vi "Track_overlay_draw_speed_test.vi"() -> ()   [LabVIEW 2018]
uses:
  <userlib>/_OpenG.lib/numeric/numeric.llb/Random Number Within Range - DBL__ogtk.vi
  Tracker.lvlib
panel:
  in  "Multiline grouping":i32=100
  out "Seconds per hour Image":dbl
  out "Image":picture
  in  "Background color Image":u32(colorbox)=13816530
  in  "Every N samples to merge":i32=2500
  out "Seconds per hour IMAQdx":dbl
  out "Image":T1(plugin-control)
  out "Error Out":errorcluster
  in  "Error In":errorcluster
  in  "Background color":u32(colorbox)=13816530
  in  "Track length, seconds (@100 fps)":i32=10
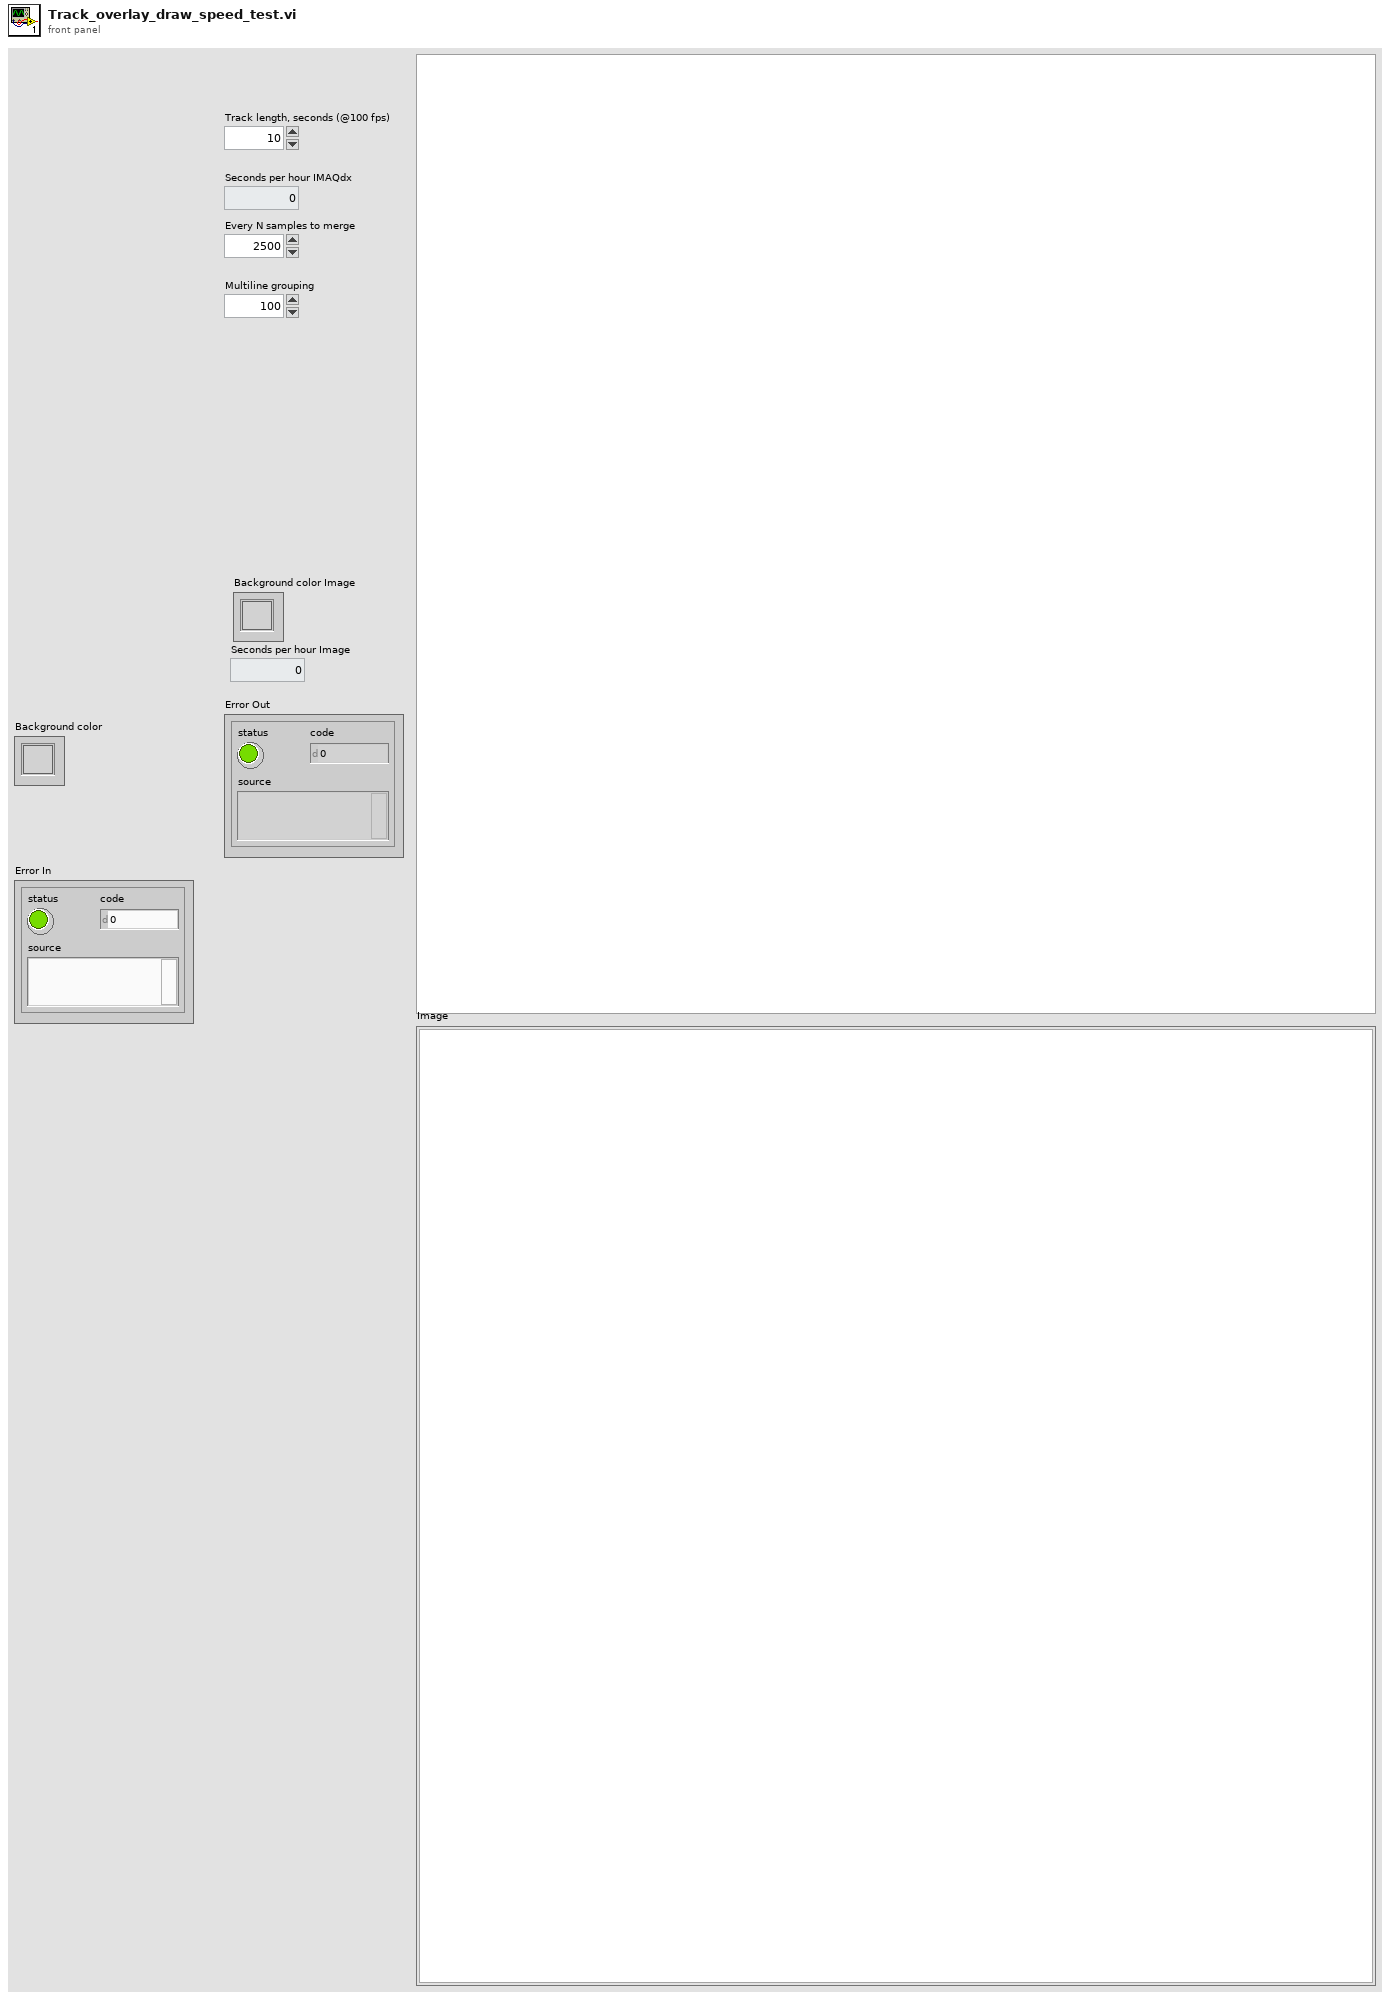
[diagram p1: front panel]
types:
  T1 = typedef "IMAQ Image.ctl" = refnum<image>
  T2 = cluster{"Left":i32, "Top":i32, "Right":i32, "Bottom":i32}
  T3 = typedef "Image Type" = u32
  T4 = cluster{"Random Number":dbl, "Random Number":dbl}
  T5 = cluster{"Random Number":dbl, "Random Number":dbl}[]
  T6 = cluster{"Width":u16, "Style":enum32{"Solid", "Dash", "Dot", "DashDot", "DashDotDot"}}
  T7 = typedef "imagedata.ctl" = cluster{"image type":i32, "image depth":i32, "image":u8[], "mask":u8[], "colors":u32[], "Rectangle":cluster{"left":i16, "top":i16, "right":i16, "bottom":i16}}
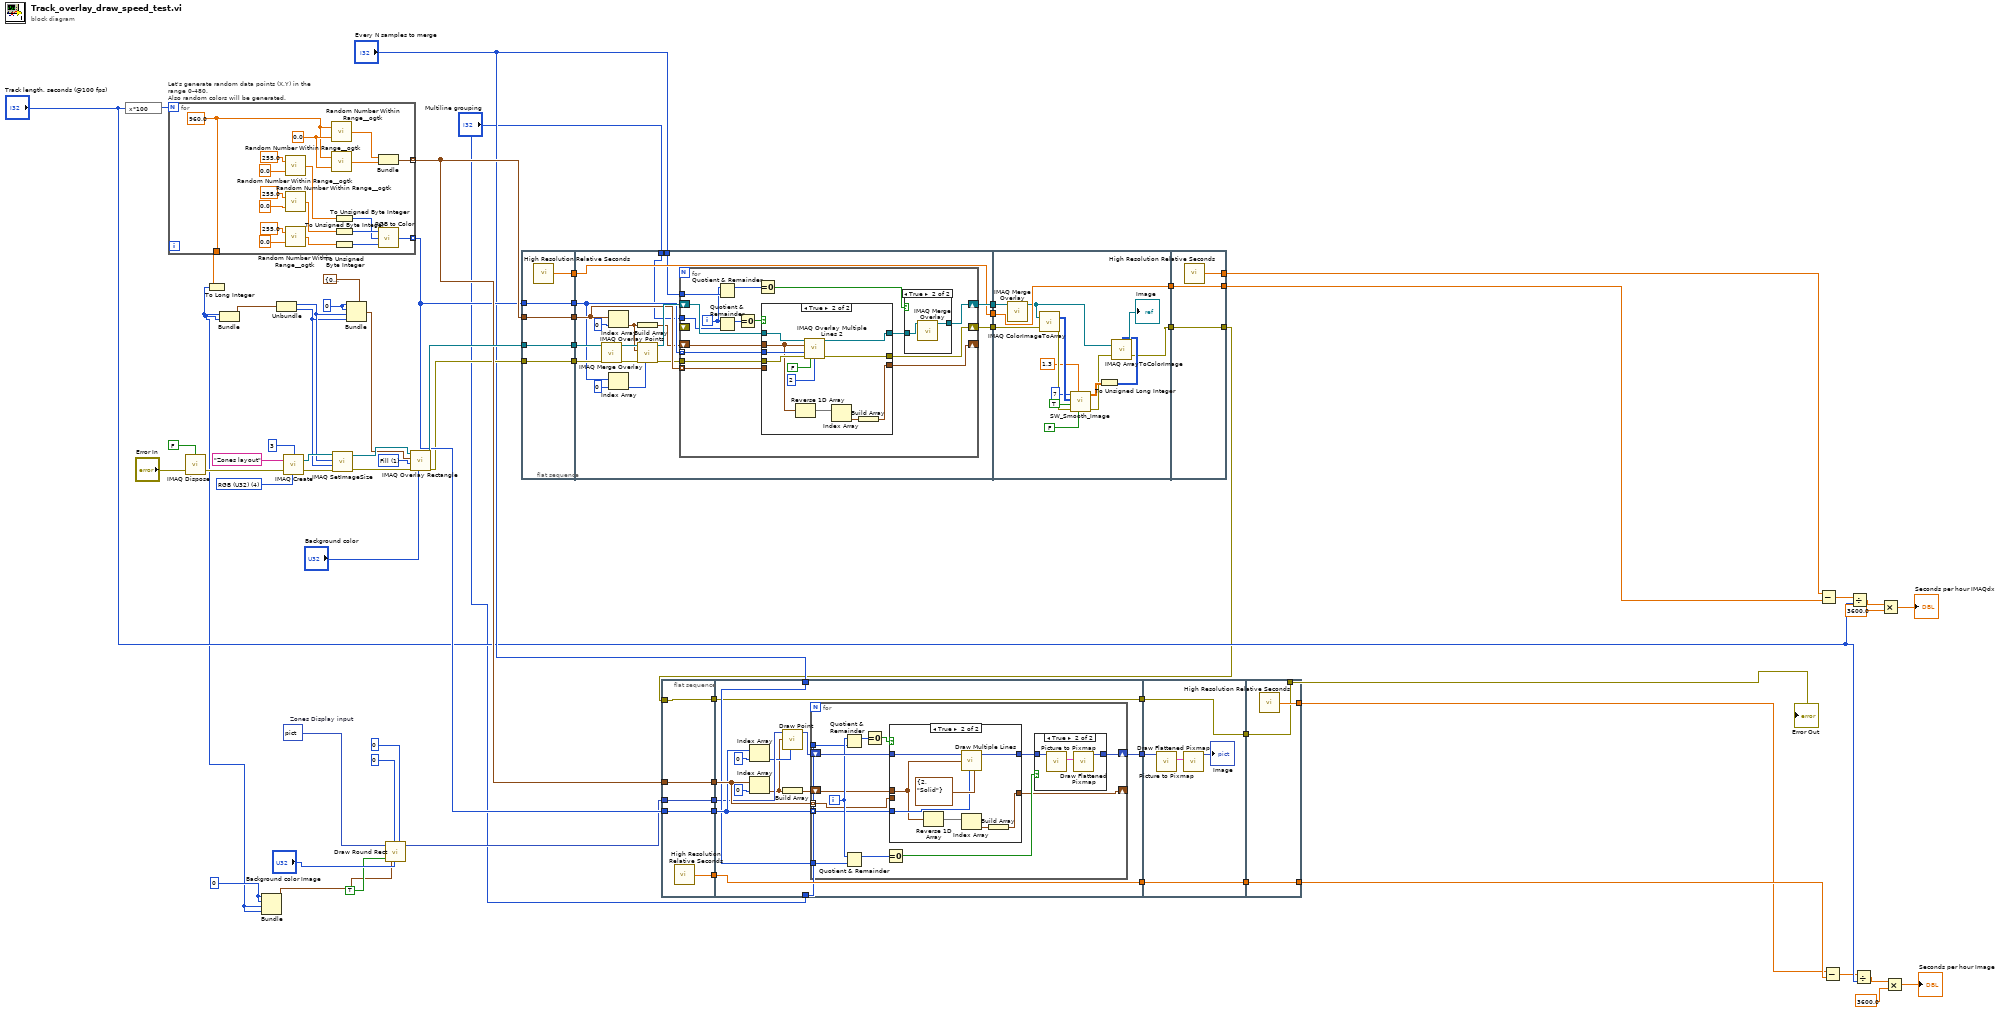
[diagram p0: block diagram]
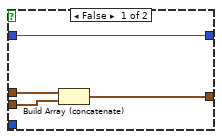
[diagram p2: hidden frame]
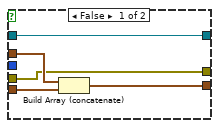
[diagram p4: hidden frame]
diagram:
  w2 = 0
  w50 = picture data[5B]  # Zones Display input
  w57 = 0 ("Left")
  w62 = u32 1 items=["Frame", "Fill", "Highlight"] ("Drawing Mode (Frame)")
  w67 = T3 4 items=["Grayscale (U8)", "Grayscale (I16)", "Grayscale (SGL)", "Complex (CSG)", "RGB (U32)", "HSL (U32)", "RGB (U64)", "Grayscale (U16)"] ("Image Type")
  n1 = expression code="x*100"("Track length, seconds (@100 fps)") -> (w70:i32)
  n2 = for "Let's generate random data points (X,Y) in the range 0-480.\nAlso random colors will be generated." {
    N: w70 -> [_]
    tunnel: [w86] -> w46 mode=indexing
    tunnel: [w72] -> w45 mode=indexing
    tunnel: [w71] -> w4
    w85 = 0.0 ("Low")
    w71 = 960.0 ("High")
    n3 = call-poly <userlib>:"Random Number Within Range__ogtk.vi"("High"=255.0, "Low"=0.0) -> ("Random Number"=w81:dbl)  [unwired: 3 in]
    n4 = call-poly <userlib>:"Random Number Within Range__ogtk.vi"("High"=255.0, "Low"=0.0) -> ("Random Number"=w80:dbl)  [unwired: 3 in]
    n5 = call-poly <userlib>:"Random Number Within Range__ogtk.vi"("High"=255.0, "Low"=0.0) -> ("Random Number"=w74:dbl)  [unwired: 3 in]
    n6 = call-poly <userlib>:"Random Number Within Range__ogtk.vi"("High"=w71, "Low"=w85) -> ("Random Number"=w88:dbl)  [unwired: 3 in]
    n7 = call-poly <userlib>:"Random Number Within Range__ogtk.vi"("High"=w71, "Low"=w85) -> ("Random Number"=w87:dbl)  [unwired: 3 in]
    n8 = To Unsigned Byte Integer(number=w81) -> (unsigned 8bit integer=w82:u8)
    n9 = To Unsigned Byte Integer(number=w80) -> (unsigned 8bit integer=w77:u8)
    n10 = To Unsigned Byte Integer(number=w74) -> (unsigned 8bit integer=w73:u8)
    n11 = Bundle("Random Number"=w88, "Random Number"=w87) -> (w86:T4)  [unwired: 1 in]
    n12 = call <vilib>:"RGB to Color.vi"("B"=w73, "G"=w77, "R"=w82) -> ("Color"=w72:u32)
  }
  n13 = call "IMAQ Dispose"("All Images? (No)"=FALSE, "error in (no error)"="Error In") -> ("error out"=w53:errorcluster)  [unwired: 4 in]
  n14 = To Long Integer(number=w4) -> (32bit integer=w1:i32)
  n15 = Bundle(w1, w1) -> (w5:cluster{i32, i32})  [unwired: 1 in]
  n16 = Bundle(w2, w2, w1, w1) -> (w3:cluster{i32, i32, i32, i32})  [unwired: 1 in]
  n17 = Unbundle(w5) -> (w59:i32, w58:i32)
  n18 = call "IMAQ Create"("Border Size"=3, "Image Name"="Zones layout", "Image Type"=w67, "error in (no error)"=w53) -> ("New Image"=w65:T1, "error out"=w66:errorcluster)  [unwired: 1 in]
  n19 = call "IMAQ SetImageSize"("error in (no error)"=w66, "Y Resolution"=w58, "X Resolution"=w59, "Image"=w65) -> ("error out"=w64:errorcluster, "Image Out"=w63:T1)  [unwired: 1 in]
  n20 = Bundle(cluster=T2 {"Left"=0, "Top"=0, "Right"=480, "Bottom"=480} ("Rectangle"), "Left"=w57, "Top"=w57, "Right"=w59, "Bottom"=w58) -> (w60:T2)
  n21 = call <vilib>:"Draw Round Rect.vi"("picture"=w50, "oval width"=i16 0, "rect"=w3, "fill?(F)"=TRUE, "color(black)"="Background color Image", "oval height"=i16 0) -> ("new picture"=w42:picture)  [unwired: 3 in]
  n22 = call "IMAQ Overlay Rectangle"("Color"="Background color", "error in (no error)"=w64, "Drawing Mode (Frame)"=w62, "Rectangle"=w60, "Image"=w63) -> ("error out"=w44:errorcluster, "Image Out"=w56:T1)  [unwired: 5 in]
  n23 = flat-sequence {
    tunnel: w45 -> [w90]
    tunnel: w46 -> [w91]
    tunnel: w44 -> [w92]
    tunnel: w56 -> [w93]
    tunnel: [w93] -> w27
    tunnel: [w92] -> w26
    tunnel: [w91] -> w25
    tunnel: [w90] -> w24
    tunnel: [w89] -> w23
    tunnel: w27 -> [w111]
    tunnel: w26 -> [w110]
    tunnel: w25 -> [w103]
    tunnel: w24 -> [w102]
    tunnel: [w101] -> w22
    tunnel: [w100] -> w21
    tunnel: [w99] -> w20
    tunnel: w23 -> [w99]
    tunnel: "Every N samples to merge" -> [w98]
    tunnel: "Multiline grouping" -> [w94]
    tunnel: w22 -> [w160]
    tunnel: w21 -> [w159]
    tunnel: w20 -> [w161]
    tunnel: [w151] -> w19
    tunnel: [w161] -> w18
    tunnel: [w162] -> w40
    tunnel: [w163] -> w39
    tunnel: [w164] -> w10
    tunnel: w19 -> [w164]
    tunnel: w18 -> [w163]
    frame #0 {
      n24 = call <vilib>:"High Resolution Relative Seconds.vi"() -> ("relative seconds"=w89:dbl)
    }
    frame #1 {
      n25 = call "IMAQ Merge Overlay"("error in (no error)"=w110, "Image Src"=w111) -> ("error out"=w105:errorcluster, "Image Dst Out"=w107:T1)  [unwired: 8 in]
      n26 = Index Array(array=w103, index=0) -> (element=w97:T4)
      n27 = Index Array(array=w102, index=0) -> (element=w106:u32)
      n28 = Build Array(w97) -> (w96:T5)
      n29 = call "IMAQ Overlay Points"("Color"=w106, "error in (no error)"=w105, "Point"=w97, "Image"=w107) -> ("error out"=w95:errorcluster, "Image Out"=w104:T1)  [unwired: 6 in]
      n30 = for {
        shift-right: [w126] -> w101
        shift-left: w104 -> [w117]
        tunnel: w103 -> [w123] mode=indexing
        tunnel: w102 -> [w121] mode=indexing
        shift-right: [w118] -> w100
        shift-left: _ -> [_]
        tunnel: w98 -> [w124]
        shift-right: [w116] -> _
        shift-left: w96 -> [w122]
        tunnel: w95 -> [w120]
        tunnel: w94 -> [w112]
        i -> [w113]
        n31 = Quotient & Remainder(x=w113, y=w124) -> (x-y*floor(x/y)=w125:i32)  [unwired: 1 out]
        n32 = Quotient & Remainder(x=w113, y=w112) -> (x-y*floor(x/y)=w115:i32)  [unwired: 1 out]
        n33 = Equal To 0?(x=w115) -> (x = 0?=w114:bool)
        n34 = Equal To 0?(x=w125) -> (x = 0?=w127:bool)
        n35 = case shown="True" w114 {
          tunnel: w123 -> [w129 _]
          tunnel: w122 -> [w131 w137]
          tunnel: w121 -> [_ w143]
          tunnel: w120 -> [w128 w142]
          tunnel: [w132 w141] -> w119
          tunnel: [w128 w140] -> w118
          tunnel: w117 -> [w132 w139]
          tunnel: [w130 w134] -> w116
          frame False {
            n36 = Build Array (concatenate)(w131, w129) -> (w130:T5)
          }
          frame True {
            n37 = Reverse 1D Array(array=w137) -> (reversed array=w136:T5)
            n38 = call "IMAQ Overlay Multiple Lines 2"("Image"=w139, "Line End Points"=w137, "Color"=w143, "error in (no error)"=w142, "Maintain Width?"=FALSE, "Width"=u32 2) -> ("Image Out"=w141:T1, "error out"=w140:errorcluster)  [unwired: 8 in]
            n39 = Index Array(array=w136) -> (element=w135:T4)  [unwired: 1 in]
            n40 = Build Array(w135) -> (w134:T5)
          }
        }
        n41 = case shown="True" w127 {
          tunnel: w119 -> [w144 w146]
          tunnel: [w144 w145] -> w126
          frame False {
          }
          frame True {
            n42 = call "IMAQ Merge Overlay"("Image Src"=w146) -> ("Image Dst Out"=w145:T1)  [unwired: 9 in, 1 out]
          }
        }
      }
    }
    frame #2 {
      n43 = call "IMAQ Merge Overlay"("Image Src"=w160) -> ("Image Dst Out"=w154:T1)  [unwired: 9 in, 1 out]
      n44 = call "IMAQ ColorImageToArray"("Image"=w154, "error in (no error)"=w159) -> ("Image Pixels (U32)"=w158:u32[][], "error out"=w157:errorcluster)  [unwired: 2 in, 1 out]
      n45 = call "SW_Smooth_Image.vi"("Normalize to 8-bit range? (T)"=FALSE, "Sigma"=1.3, "Error In"=w157, "Image? (T)"=TRUE, "Array or pixmap in"=w158, "Kernel size"=u32 7) -> ("Error Out"=w152:errorcluster, "Array or pixmap out"=w156:dbl[][])  [unwired: 4 in]
      n46 = To Unsigned Long Integer(number=w156) -> (unsigned 32bit integer=w153:u32[][])
      n47 = call "IMAQ ArrayToColorImage"("Image Pixels (U32)"=w153, "Image"=w154, "error in (no error)"=w152) -> ("Image Out"=→"Image":T1, "error out"=w151:errorcluster)  [unwired: 2 in]
    }
    frame #3 {
      n48 = call <vilib>:"High Resolution Relative Seconds.vi"() -> ("relative seconds"=w162:dbl)
    }
  }
  n49 = flat-sequence {
    tunnel: w45 -> [w167]
    tunnel: w46 -> [w168]
    tunnel: w42 -> [w169]
    tunnel: [w169] -> w17
    tunnel: [w168] -> w16
    tunnel: [w167] -> w15
    tunnel: [w166] -> w14
    tunnel: w10 -> [w165]
    tunnel: [w165] -> w6
    tunnel: w17 -> [w176]
    tunnel: w16 -> [w181]
    tunnel: w15 -> [w180]
    tunnel: [w179] -> w13
    tunnel: [w178] -> w12
    tunnel: w14 -> [w178]
    tunnel: "Every N samples to merge" -> [w177]
    tunnel: "Multiline grouping" -> [w175]
    tunnel: [w170] -> w7
    tunnel: w6 -> [w170]
    tunnel: w13 -> [w216]
    tunnel: w12 -> [w218]
    tunnel: [w218] -> w11
    tunnel: [w214] -> w8
    tunnel: w7 -> [w214]
    tunnel: [w220] -> w29
    tunnel: [w221] -> w30
    tunnel: w11 -> [w221]
    tunnel: [w219] -> w9
    tunnel: w8 -> [w219]
    frame #0 {
      n50 = call <vilib>:"High Resolution Relative Seconds.vi"() -> ("relative seconds"=w166:dbl)
    }
    frame #1 {
      n51 = Index Array(array=w180, index=0) -> (element=w173:u32)
      n52 = Index Array(array=w181, index=0) -> (element=w172:T4)
      n53 = call <vilib>:"Draw Point.vi"("picture"=w176, "point(x,y)"=w172, "color(black)"=w173) -> ("new picture"=w174:picture)  [unwired: 6 in]
      n54 = Build Array(w172) -> (w171:T5)
      n55 = for {
        shift-right: [w194] -> w179
        shift-left: w174 -> [w193]
        tunnel: w181 -> [w188] mode=indexing
        tunnel: w180 -> [w185] mode=indexing
        tunnel: w177 -> [w195]
        tunnel: w175 -> [w190]
        shift-right: [w186] -> _
        shift-left: w171 -> [w187]
        i -> [w191]
        n56 = Quotient & Remainder(x=w191, y=w190) -> (x-y*floor(x/y)=w192:i32)  [unwired: 1 out]
        n57 = Quotient & Remainder(x=w191, y=w195) -> (x-y*floor(x/y)=w196:i32)  [unwired: 1 out]
        n58 = Equal To 0?(x=w192) -> (x = 0?=w184:bool)
        n59 = Equal To 0?(x=w196) -> (x = 0?=w197:bool)
        n60 = case shown="True" w184 {
          tunnel: w193 -> [w201 w204]
          tunnel: [w201 w203] -> w189
          tunnel: w188 -> [w200 _]
          tunnel: w187 -> [w199 w205]
          tunnel: [w198 w202] -> w186
          tunnel: w185 -> [_ w206]
          frame False {
            n61 = Build Array (concatenate)(w199, w200) -> (w198:T5)
          }
          frame True {
            n62 = Reverse 1D Array(array=w205) -> (reversed array=w209:T5)
            n63 = call <vilib>:"Draw Multiple Lines.vi"("picture"=w204, "line endpoints"=w205, "color(black)"=w206, "pen"=T6 {"Width"=2, "Style"=enum."Solid"}) -> ("new picture"=w203:picture)  [unwired: 5 in]
            n64 = Index Array(array=w209) -> (element=w208:T4)  [unwired: 1 in]
            n65 = Build Array(w208) -> (w202:T5)
          }
        }
        n66 = case shown="True" w197 {
          tunnel: [w210 w212] -> w194
          tunnel: w189 -> [w210 w211]
          frame False {
          }
          frame True {
            n67 = call <vilib>:"Picture to Pixmap.vi"("picture"=w211) -> ("image data"=w213:T7)  [unwired: 9 in, 1 out]
            n68 = call <vilib>:"Draw Flattened Pixmap.vi"("image data"=w213) -> ("new picture"=w212:picture)  [unwired: 8 in]
          }
        }
      }
    }
    frame #2 {
      n69 = call <vilib>:"Picture to Pixmap.vi"("picture"=w216) -> ("image data"=w217:T7)  [unwired: 9 in, 1 out]
      n70 = call <vilib>:"Draw Flattened Pixmap.vi"("image data"=w217) -> ("new picture"=→"Image":picture)  [unwired: 8 in]
    }
    frame #3 {
      n71 = call <vilib>:"High Resolution Relative Seconds.vi"() -> ("relative seconds"=w220:dbl)
    }
  }
  n72 = Subtract(x=w40, y=w39) -> (x-y=w38:dbl)
  n73 = Subtract(x=w29, y=w30) -> (x-y=w31:dbl)
  n74 = Divide(x=w38, y="Track length, seconds (@100 fps)") -> (x/y=w37:dbl)
  n75 = Divide(x=w31, y="Track length, seconds (@100 fps)") -> (x/y=w32:dbl)
  n76 = Multiply(x=w37, y=3600.0) -> (x*y=→"Seconds per hour IMAQdx":dbl)
  n77 = Multiply(x=w32, y=3600.0) -> (x*y=→"Seconds per hour Image":dbl)
  "Error Out" <- w9
